vi "Set Current (SubVI).vi"(9 "current(A)":dbl, 10 "freq":dbl, 11 "队列输入":refnum<queue>) -> ()   [LabVIEW 2019, in "SubVI.lvlib"]
uses:
  SubVI.lvlib
  config.ctl
  Instrument.ctl
  lib/QDInstrument.dll
  <vilib>/NI/Modbus Library/API/Master/Modbus Master.lvclass
panel:
  # "(真是通道1，假是通道2)"
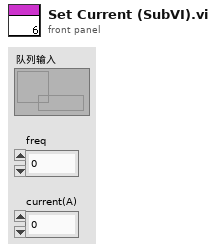
[diagram p1: front panel]
types:
  T1 = typedef "config.ctl" = cluster{"initialize":string, "6221":cluster{"6221 Resource":refnum<visa-resource-name>, "Delta status":bool}, "7001":cluster{"Ch":bool}, "SR830+6221":cluster{"source":u16, "阻抗":dbl, "量程入 4":i32, "量程入 3":i32, "量程入 2":i32, "量程入 1":i32, "电流":dbl, "SR830 2":bool, "SR830 3":bool, "SR830 4":bool, "SR830 1":bool, "VISA 1":refnum<visa-resource-name>, "VISA 2":refnum<visa-resource-name>, "VISA 3":refnum<visa-resource-name>, "VISA 4":refnum<visa-resource-name>, "量程":enum16{"量程每次测量会判定", "量程不变为设定值"}}, "2400":cluster{"2400":bool, "VISA":refnum<visa-resource-name>}, "ch":cluster{"ch str":string, "ch1":bool, "ch2":bool, "布尔":bool}, "error":bool, "数据文件路径":path, "log":cluster{"log路径":path, "log interval":dbl}, "Instrument":T2}
  T2 = typedef "Instrument.ctl" = cluster{"335 Resource":refnum<visa-resource-name>, "Input (0:A)":u16, "Instrument Type":i32, "quantum design":refnum<k24>, "Heater Output (1:1)":u16, "335state":refnum<vi>, "semaphore":T3, "TCP master instance":refnum<class "Modbus Master.lvclass">}
  T3 = typedef "Semaphore RefNum" = refnum<k1>
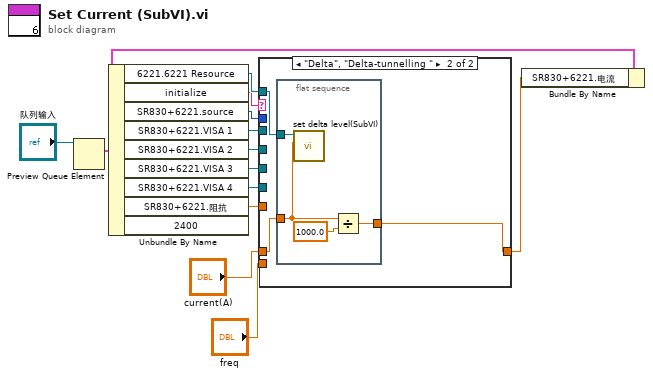
[diagram p0: block diagram]
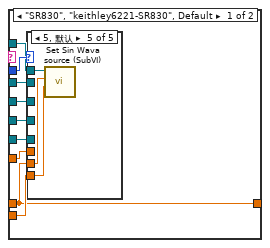
[diagram p2: hidden frame]
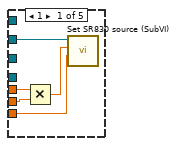
[diagram p3: hidden frame]
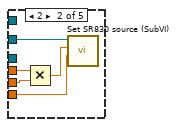
[diagram p4: hidden frame]
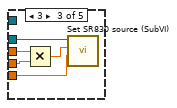
[diagram p5: hidden frame]
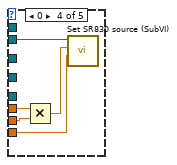
[diagram p6: hidden frame]
diagram:
  n1 = Preview Queue Element(queue="队列输入") -> (element=w10:T1)  [unwired: 2 in, 3 out]
  n2 = Unbundle By Name(w10) -> ("6221.6221 Resource"=w2:refnum<visa-resource-name>, "initialize"=w1:string, "SR830+6221.source"=w4:u16, "SR830+6221.VISA 1"=w5:refnum<visa-resource-name>, "SR830+6221.VISA 2"=w6:refnum<visa-resource-name>, "SR830+6221.VISA 3"=w7:refnum<visa-resource-name>, "SR830+6221.VISA 4"=w8:refnum<visa-resource-name>, "SR830+6221.阻抗"=w9:dbl)  [unwired: 1 out]
  n3 = case shown="\"Delta\", \"Delta-tunnelling \"" w1 {
    tunnel: w2 -> [w20 w47]
    tunnel: "current(A)" -> [w14 w48]
    tunnel: w4 -> [w22 _]
    tunnel: "freq" -> [w21 _]
    tunnel: w5 -> [w19 _]
    tunnel: w6 -> [w18 _]
    tunnel: w7 -> [w17 _]
    tunnel: w8 -> [w16 _]
    tunnel: w9 -> [w15 _]
    tunnel: [w14 w46] -> w11
    frame "SR830", "keithley6221-SR830", Default {
      n4 = case shown="5, 默认" w22 {
        tunnel: w21 -> [w23 w28 w33 w38 w45]
        tunnel: w19 -> [_ _ _ w41 _]
        tunnel: w16 -> [_ _ w36 _ _]
        tunnel: w17 -> [_ w31 _ _ _]
        tunnel: w18 -> [w26 _ _ _ _]
        tunnel: w20 -> [_ _ _ _ w44]
        tunnel: w14 -> [w24 w29 w35 w40 w43]
        tunnel: w15 -> [w27 w32 w37 w42 _]
        frame 1 {
          n5 = Multiply(x=w27, y=w24) -> (x*y=w25:dbl)
          n6 = call "Set SR830 source (SubVI).vi"("freq"=w23, "voltage"=w25, "VISA引用句柄输入"=w26) -> ()  [unwired: 9 in]
        }
        frame 2 {
          n7 = Multiply(x=w32, y=w29) -> (x*y=w30:dbl)
          n8 = call "Set SR830 source (SubVI).vi"("freq"=w28, "voltage"=w30, "VISA引用句柄输入"=w31) -> ()  [unwired: 9 in]
        }
        frame 3 {
          n9 = Multiply(x=w37, y=w35) -> (x*y=w34:dbl)
          n10 = call "Set SR830 source (SubVI).vi"("freq"=w33, "voltage"=w34, "VISA引用句柄输入"=w36) -> ()  [unwired: 9 in]
        }
        frame 0 {
          n11 = Multiply(x=w42, y=w40) -> (x*y=w39:dbl)
          n12 = call "Set SR830 source (SubVI).vi"("freq"=w38, "voltage"=w39, "VISA引用句柄输入"=w41) -> ()  [unwired: 9 in]
        }
        frame 5, Default {
          n13 = call "Set Sin Wava source (SubVI).vi"("Hz"=w45, "A"=w43, "VISA引用句柄输入"=w44) -> ()  [unwired: 9 in]
        }
      }
    }
    frame "Delta", "Delta-tunnelling " {
      n14 = flat-sequence {
        tunnel: [w49] -> w46
        tunnel: w47 -> [w52]
        tunnel: w48 -> [w51]
        frame #0 {
          n15 = call "set delta level(SubVI).vi"("电流（A）"=w51, "VISA引用句柄输入"=w52) -> ()  [unwired: 8 in, 2 out]
          n16 = Divide(x=w51, y=1000.0) -> (x/y=w49:dbl)
        }
      }
    }
  }
  n17 = Bundle By Name(cluster=w10, "SR830+6221.电流"=w11) -> ()  [unwired: 1 out]
